vi "ReadIO.one.loop.fpga.vi"(8 "Channel":u32, 9 "Delta time":u32, 10 "Number of time points":i32, 11 "Memory (in)":refnum<k21>="InputMatrix") -> ()   [LabVIEW 2012]
uses:
  <vilib>/rvi/eio/common/nirviEmuTemplateMethod_errors.vi
  <vilib>/rvi/DataTransferAndStorage/Container/Common/niFpgaContainerExecOnDevCompGetState.vi
  <vilib>/rvi/DataTransferAndStorage/Container/Common/niFpgaContainerGetUniqueNameForEmu.vi
  <vilib>/rvi/Memory/Memory_Emulation/niFpgaMemoryEmulationCacheClearOnFirstRun.vi
  <vilib>/rvi/Memory/Memory_Emulation/nirvimemoryEmulationManagerCache_MakeExclusive.vi
  <vilib>/rvi/Memory/Memory_Emulation/niFpgaMemoryEmulationValidateCache.vi
  <vilib>/rvi/Memory/Memory_Emulation/nirvimemoryEmulationManagerCache_ReleaseExclusive.vi
  <vilib>/rvi/Memory/Memory_Emulation/nirvimemoryEmulationManagerCache_InsertValue.vi
  <vilib>/Utility/error.llb/Clear Errors.vi
  <vilib>/rvi/Emulation/niFpgaSctlEmulationGetInTimedLoop.vi
  <vilib>/rvi/Memory/Memory_Emulation/nirvimemoryEmulationManagerCache_GetValue.vi
  <vilib>/rvi/Memory/Memory_Emulation/nirvimemoryEmulationManagerCache_SetValue.vi
  <vilib>/rvi/Emulation/niFpgaSctlEmulationResourceMgr.vi
  <vilib>/eio/EIONode/EIONode.xnode
  <vilib>/rvi/DataTransferAndStorage/Container/XNode/niFpgaContainer.xnode
  <vilib>/rvi/Memory/Memory_Emulation/niFpgaMemoryEmulationRefIn.vi
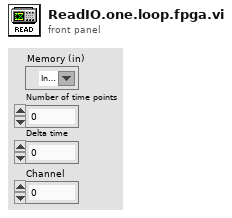
[diagram p1: front panel]
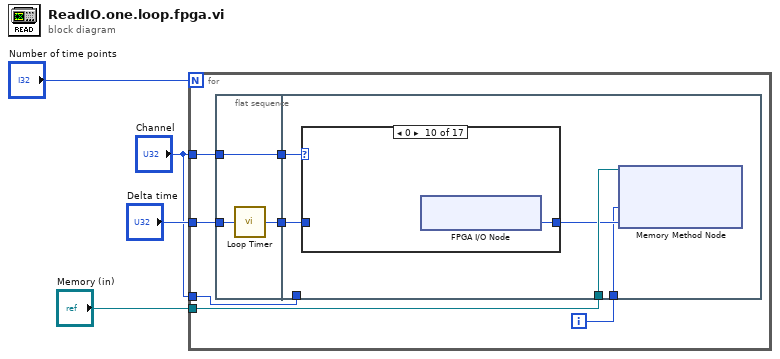
[diagram p0: block diagram]
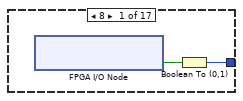
[diagram p2: hidden frame]
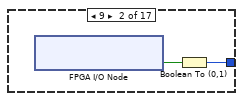
[diagram p3: hidden frame]
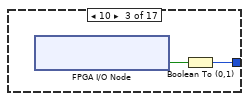
[diagram p4: hidden frame]
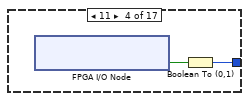
[diagram p5: hidden frame]
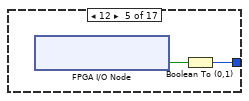
[diagram p6: hidden frame]
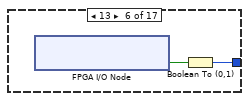
[diagram p7: hidden frame]
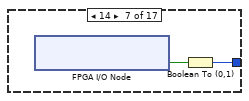
[diagram p8: hidden frame]
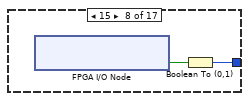
[diagram p9: hidden frame]
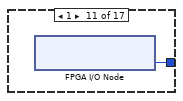
[diagram p11: hidden frame]
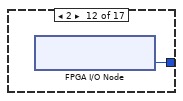
[diagram p12: hidden frame]
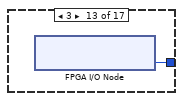
[diagram p13: hidden frame]
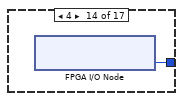
[diagram p14: hidden frame]
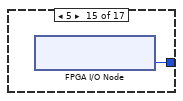
[diagram p15: hidden frame]
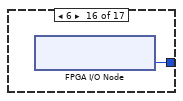
[diagram p16: hidden frame]
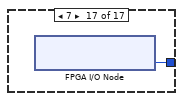
[diagram p17: hidden frame]
diagram:
  n1 = for {
    N: "Number of time points" -> [_]
    tunnel: "Delta time" -> [w11]
    tunnel: "Memory (in)" -> [w10]
    tunnel: "Channel" -> [w8]
    tunnel: "Channel" -> [w6]
    i -> [w9]
    n2 = flat-sequence {
      tunnel: w11 -> [w14]
      tunnel: [w13] -> w7
      tunnel: w6 -> [w13]
      tunnel: [w12] -> w5
      tunnel: w10 -> [w19]
      tunnel: w9 -> [w16]
      tunnel: w8 -> [_]
      tunnel: w7 -> [w18]
      tunnel: w5 -> [w15]
      frame #0 {
        n3 = call "Loop Timer"("Count(Ticks)"=w14) -> ("Tick Count(Ticks)"=w12:u32)
      }
      frame #1 {
        n4 = case shown="0" w18 {
          tunnel: [w21 w22 w24 w26 w28 w30 w32 w34 w36 w37 w38 w39 w40 w41 w42 w43 w44] -> w17
          tunnel: w15 -> [_ _ _ _ _ _ _ _ w36 _ _ _ _ _ _ _ _]
          frame 8 {
            n5 = xnode "FPGA I/O Node"() -> ("Connector0/DIO8"=w20:bool)  [unwired: 1 in, 1 out]
            n6 = Boolean To (0,1)(Boolean=w20) -> (0, 1=w21:i16)
          }
          frame 9 {
            n7 = xnode "FPGA I/O Node"() -> ("Connector0/DIO9"=w23:bool)  [unwired: 1 in, 1 out]
            n8 = Boolean To (0,1)(Boolean=w23) -> (0, 1=w22:i16)
          }
          frame 10 {
            n9 = xnode "FPGA I/O Node"() -> ("Connector0/DIO10"=w25:bool)  [unwired: 1 in, 1 out]
            n10 = Boolean To (0,1)(Boolean=w25) -> (0, 1=w24:i16)
          }
          frame 11 {
            n11 = xnode "FPGA I/O Node"() -> ("Connector0/DIO11"=w27:bool)  [unwired: 1 in, 1 out]
            n12 = Boolean To (0,1)(Boolean=w27) -> (0, 1=w26:i16)
          }
          frame 12 {
            n13 = xnode "FPGA I/O Node"() -> ("Connector0/DIO12"=w29:bool)  [unwired: 1 in, 1 out]
            n14 = Boolean To (0,1)(Boolean=w29) -> (0, 1=w28:i16)
          }
          frame 13 {
            n15 = xnode "FPGA I/O Node"() -> ("Connector0/DIO13"=w31:bool)  [unwired: 1 in, 1 out]
            n16 = Boolean To (0,1)(Boolean=w31) -> (0, 1=w30:i16)
          }
          frame 14 {
            n17 = xnode "FPGA I/O Node"() -> ("Connector0/DIO14"=w33:bool)  [unwired: 1 in, 1 out]
            n18 = Boolean To (0,1)(Boolean=w33) -> (0, 1=w32:i16)
          }
          frame 15 {
            n19 = xnode "FPGA I/O Node"() -> ("Connector0/DIO15"=w35:bool)  [unwired: 1 in, 1 out]
            n20 = Boolean To (0,1)(Boolean=w35) -> (0, 1=w34:i16)
          }
          frame Default {
          }
          frame 0 {
            n21 = xnode "FPGA I/O Node"() -> ("Connector0/AI0"=w37:i16)  [unwired: 1 in, 1 out]
          }
          frame 1 {
            n22 = xnode "FPGA I/O Node"() -> ("Connector0/AI1"=w38:i16)  [unwired: 1 in, 1 out]
          }
          frame 2 {
            n23 = xnode "FPGA I/O Node"() -> ("Connector0/AI2"=w39:i16)  [unwired: 1 in, 1 out]
          }
          frame 3 {
            n24 = xnode "FPGA I/O Node"() -> ("Connector0/AI3"=w40:i16)  [unwired: 1 in, 1 out]
          }
          frame 4 {
            n25 = xnode "FPGA I/O Node"() -> ("Connector0/AI4"=w41:i16)  [unwired: 1 in, 1 out]
          }
          frame 5 {
            n26 = xnode "FPGA I/O Node"() -> ("Connector0/AI5"=w42:i16)  [unwired: 1 in, 1 out]
          }
          frame 6 {
            n27 = xnode "FPGA I/O Node"() -> ("Connector0/AI6"=w43:i16)  [unwired: 1 in, 1 out]
          }
          frame 7 {
            n28 = xnode "FPGA I/O Node"() -> ("Connector0/AI7"=w44:i16)  [unwired: 1 in, 1 out]
          }
        }
        n29 = xnode ("Memory Method Node")("Address"=w16, "Data"=w17, "Memory In"=w19) -> ()  [unwired: 1 out]
      }
    }
  }
